vi "Imaginary Uncertain Min Finder1.vi"(3 "output control":T3, 4 "data":T4, 5 "X":dbl[](array[numeric])) -> (0 "error out":errorcluster, 1 "gradient":dbl[](array[numeric]), 2 "f(X)":dbl)   [LabVIEW 2013]
doc: "This template is the starting point for creating an objectivel function to be passed to the Unconstrained Optimization.vi."
uses:
  <vilib>/gmath/NumericalOptimization/objective function data.ctl
  BaesDataTypeDefinition.ctl
  <vilib>/gmath/NI_Gmath.lvlib
panel:
  out "element":dbl
  in  "cluster":T2={"Imaginary or Real Part"=0.0, "Chi Square at Minimum"=0.0, "Extinction ExtinctionUncertainity Size parameter and Number ofS sizes"={"Extinction"=[], "Extinction Uncertainty"=[], "Size parameters"=[], "Number ofSizes"=0.0, "GeometricCrossSection"=[], "Wave Length"=0.0, "SMPS Sizes"=[], "Concentration"=[], "Double Charge Correction"=FALSE, "Extincation Factor"=1.0, "Diameter Factor"=1.0, "Diameter Offset"=0.0, "Extinction Factor Flag"=FALSE, "Diameter Factor Flag"=FALSE, "Diameter Offset Flag"=FALSE, "Sizes"=[], "ExtinctionOrAbsorptionOrScattering"=0, "Convergence Strength"=enum."Weak"}} {"Extinction ExtinctionUncertainity Size parameter and Number ofS sizes"."ExtinctionOrAbsorptionOrScattering" scale=0.0..2.0}
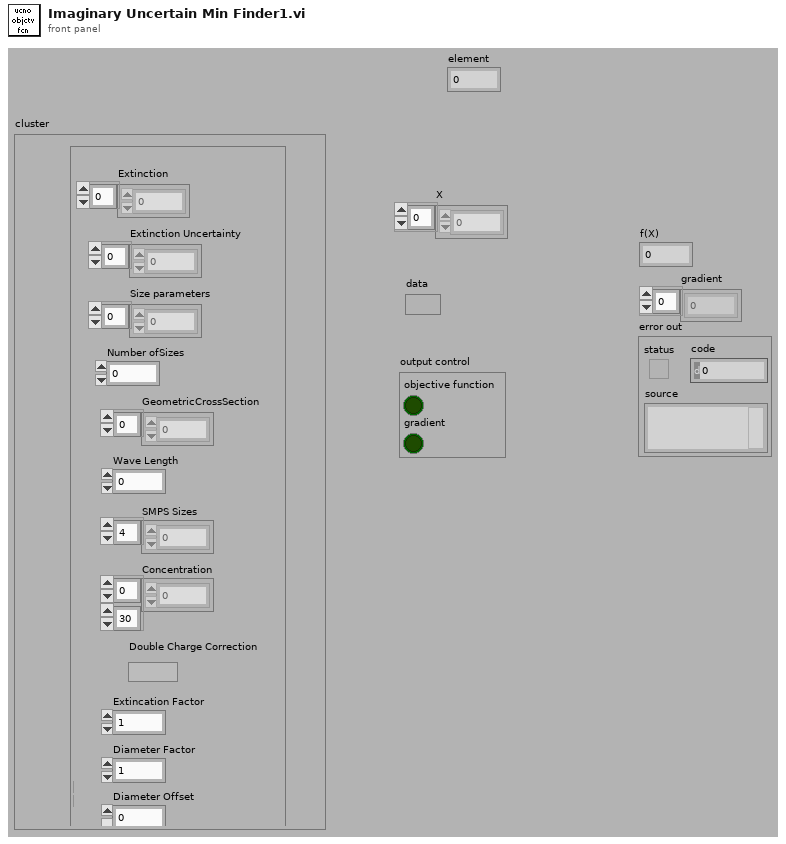
[diagram p1: front panel]
types:
  T1 = typedef "BaesDataTypeDefinition.ctl" = cluster{"Extinction":dbl[], "Extinction Uncertainty":dbl[], "Size parameters":dbl[], "Number ofSizes":dbl, "GeometricCrossSection":dbl[], "Wave Length":dbl, "SMPS Sizes":dbl[], "Concentration":dbl[][], "Double Charge Correction":bool, "Extincation Factor":dbl, "Diameter Factor":dbl, "Diameter Offset":dbl, "Extinction Factor Flag":bool, "Diameter Factor Flag":bool, "Diameter Offset Flag":bool, "Sizes":dbl[], "ExtinctionOrAbsorptionOrScattering":i8, "Convergence Strength":enum16{"Weak", "Medium", "Strong"}}
  T2 = cluster{"Imaginary or Real Part":dbl, "Chi Square at Minimum":dbl, "Extinction ExtinctionUncertainity Size parameter and Number ofS sizes":T1}
  T3 = cluster{"objective function":bool, "gradient":bool}
  T4 = typedef "NI_Gmath.lvlib/objective function data.ctl" = variant
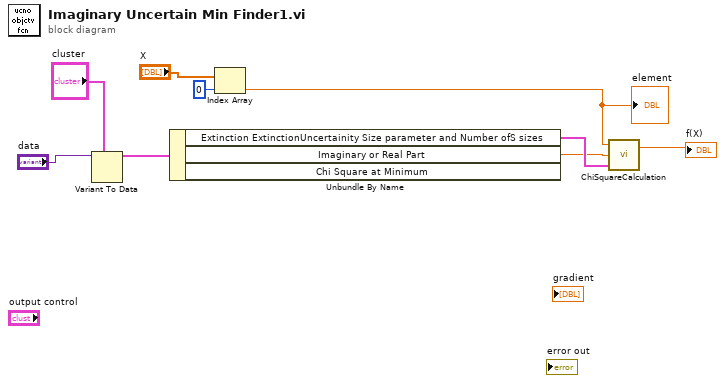
[diagram p0: block diagram]
diagram:
  n1 = Variant To Data(type="cluster", Variant="data") -> (data=w9:T2)  [unwired: 1 in, 1 out]
  n2 = Unbundle By Name(w9) -> ("Extinction ExtinctionUncertainity Size parameter and Number ofS sizes"=w4:T1, "Imaginary or Real Part"=w1:dbl)  [unwired: 1 out]
  n3 = Index Array(array="X", index=0) -> (element=w2:dbl)
  "element" <- w2
  n4 = call "ChiSquareCalculation.vi"("Extinction ExtinctionUncertainity Size parameter and Number ofS sizes 2"=w4, "refractive index, imaginary"=w1, "refractive index, real"=w2) -> ("Chi Squared"=→"f(X)":dbl)  [unwired: 1 out]
